vi "Camera_Config_Specific_Attributes.vi"(4 "Crop?":bool, 5 "Camera":T1, 6 "Detect Movement":bool, 8 "error in (no error)":errorcluster, 10 "Refnum in":T2, 11 "input cluster":T3 {"SystemVersion" items=["Standard", "XL"]; "Overlay_Ring" items=["Session Data", "Extended Setup", "Buffer", "Camera", "Dispenser", "Stats", "Connections"]; "Flush Size" min=1; "Dispense Speed" min=1; "Rectangle 2"."Rotation" format="%.2f"; "Rectangle 2"."Left" scale=0.0..1024.0; "Rectangle 2"."Right" scale=0.0..1024.0; "Rectangle 1"."Rotation" format="%.2f"; "Rectangle 1"."Left" scale=0.0..1024.0; "Rectangle 1"."Right" scale=0.0..1024.0; "Max Framerate" min=1; "Overload threshold" min=1; "Image Save Queue Size" min=1; "Image Process Queue Size" min=1; "Empty start" min=1; "Sample size threshold" min=1; "Framerate" min=1; "Light intensity" scale=0.0..100.0}) -> (0 "error out":errorcluster, 3 "Refnum out":T2)   [LabVIEW 2021]
uses:
  <vilib>/userDefined/High Color/IMAQdx.ctl
  controls/Data.ctl
  <vilib>/vision/Image Controls.llb/IMAQ Image.ctl
  Camera_ID.ctl
  <resource>/objmgr/imaqdx.rc
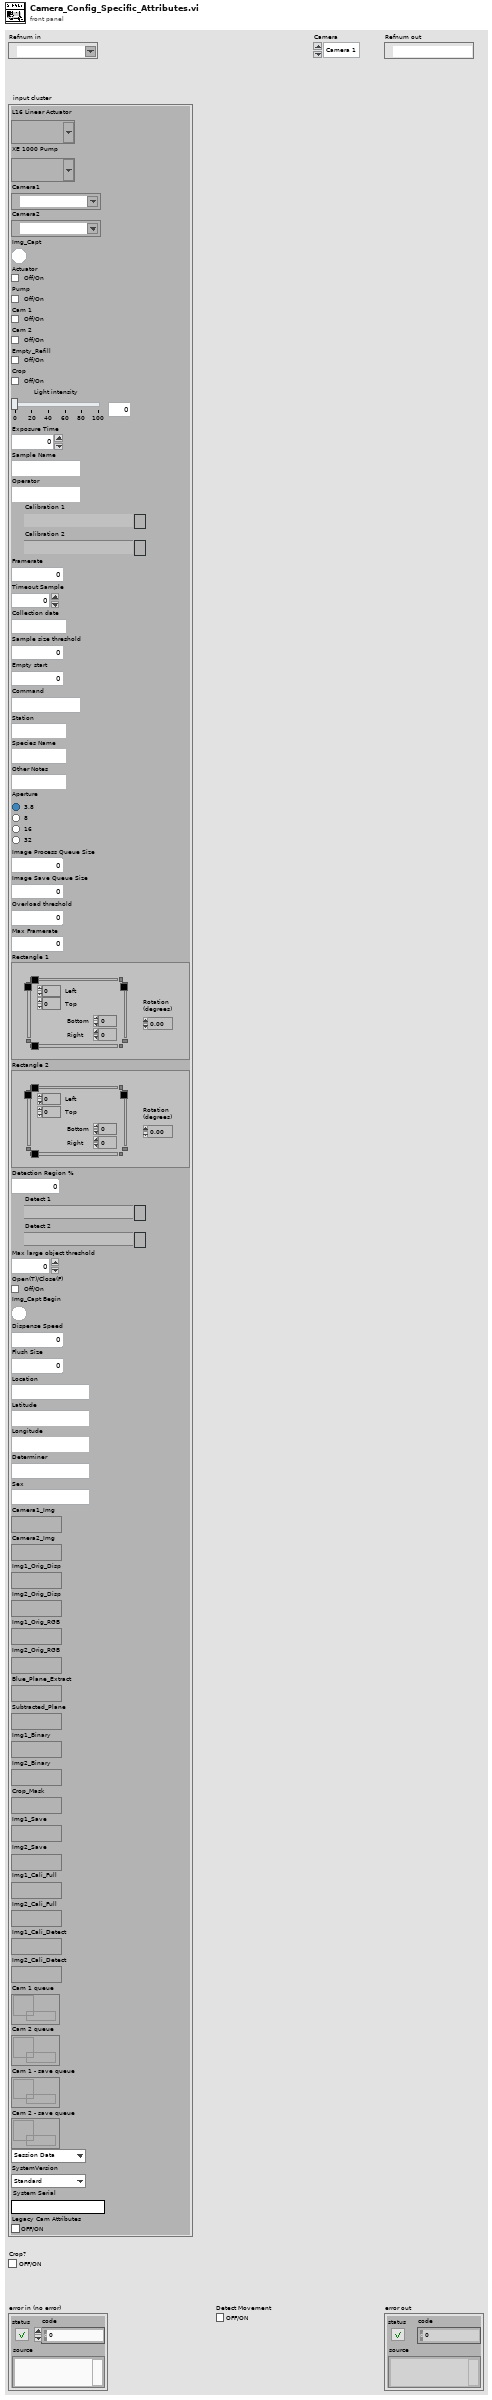
[diagram p1: front panel]
types:
  T1 = typedef "Camera_ID.ctl" = enum16{"Camera 1", "Camera 2"}
  T2 = typedef "IMAQdx.ctl" = refnum<k21>
  T3 = typedef "Data.ctl" = cluster{"L16 Linear Actuator":refnum<visa-resource-name>, "XE 1000 Pump":refnum<visa-resource-name>, "Camera1":T2, "Camera2":T2, "Img_Capt":bool, "Actuator":bool, "Pump":bool, "Cam 1":bool, "Cam 2":bool, "Empty_Refill":bool, "Crop":bool, "Light intensity":i32, "Exposure Time":dbl, "Sample Name":string, "Operator":string, "Calibration 1":path, "Calibration 2":path, "Framerate":i32, "Timeout Sample":i32, "Collection date":string, "Sample size threshold":i32, "Empty start":u32, "Command":string, "Station":string, "Species Name":string, "Other Notes":string, "Aperture":enum32{"Item 0", "Item 1", "Item 2", "Item 3"}, "Image Process Queue Size":i32, "Image Save Queue Size":i32, "Overload threshold":i32, "Max Framerate":i32, "Rectangle 1":T4, "Rectangle 2":T4, "Detection Region %":dbl, "Detect 1":path, "Detect 2":path, "Max large object threshold":i32, "Open(T)/Close(F)":bool, "Img_Capt Begin":bool, "Dispense Speed":i32, "Flush Size":i32, "Location":string, "Latitude":string, "Longitude":string, "Determiner":string, "Sex":string, "Camera1_Img":T5, "Camera2_Img":T5, "Img1_Orig_Disp":T5, "Img2_Orig_Disp":T5, "Img1_Orig_RGB":T5, "Img2_Orig_RGB":T5, "Blue_Plane_Extract":T5, "Subtracted_Plane":T5, "Img1_Binary":T5, "Img2_Binary":T5, "Crop_Mask":T5, "Img1_Save":T5, "Img2_Save":T5, "Img1_Cali_Full":T5, "Img2_Cali_Full":T5, "Img1_Cali_Detect":T5, "Img2_Cali_Detect":T5, "Cam 1 queue":refnum<queue>, "Cam 2 queue":refnum<queue>, "Cam 1 - save queue":refnum<queue>, "Cam 2 - save queue":refnum<queue>, "Overlay_Ring":u16, "SystemVersion":u16, "System Serial":string, "Legacy Cam Attributes":bool}
  T4 = typedef "IMAQ Rectangle" = cluster{"Left":i32, "Top":i32, "Right":i32, "Bottom":i32, "Rotation":dbl}
  T5 = typedef "IMAQ Image.ctl" = refnum<image>
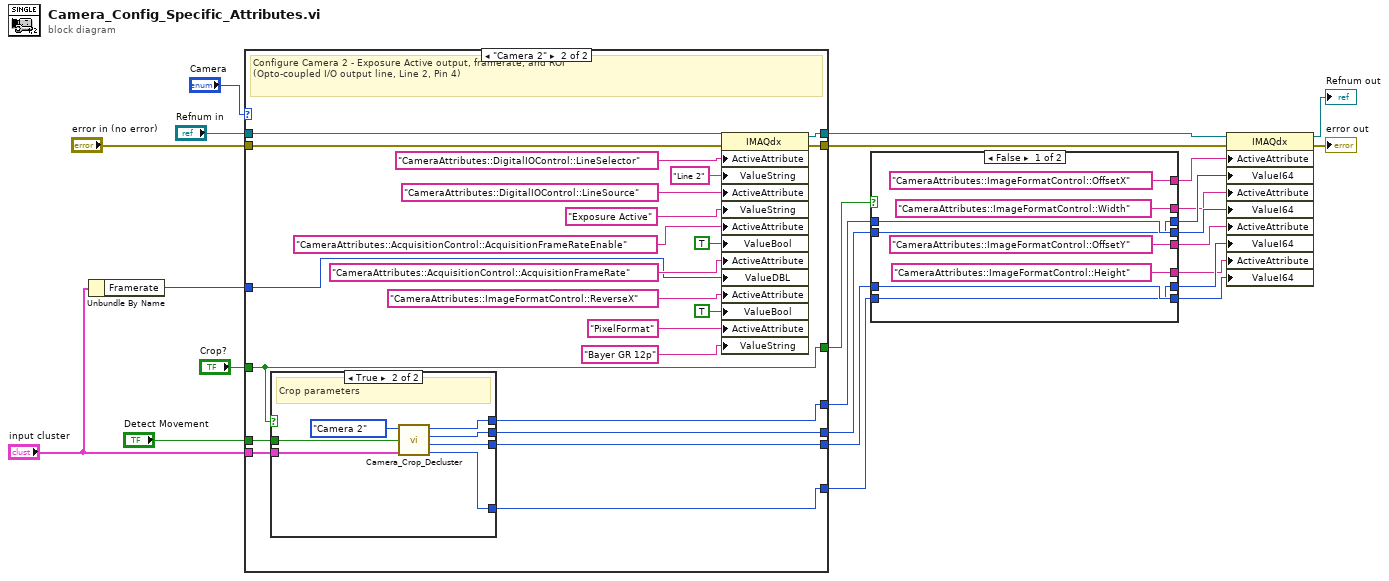
[diagram p0: block diagram]
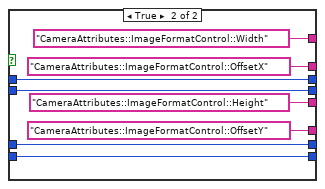
[diagram p2: hidden frame]
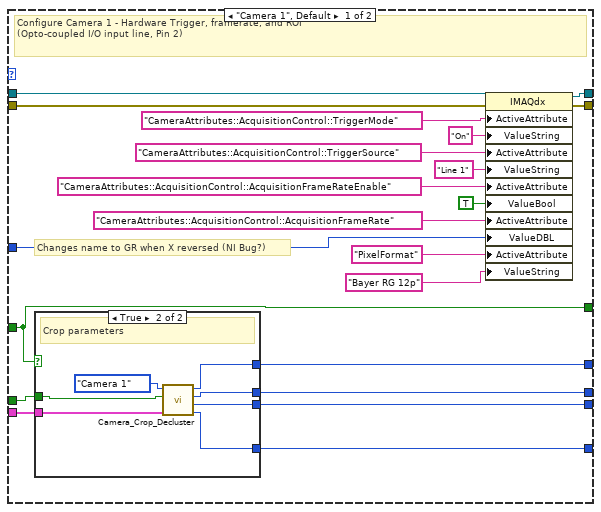
[diagram p3: hidden frame]
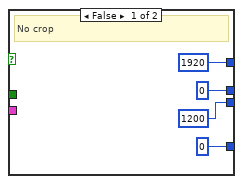
[diagram p4: hidden frame]
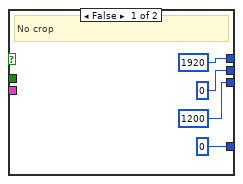
[diagram p5: hidden frame]
diagram:
  n1 = Unbundle By Name("input cluster") -> ("Framerate"=w1:i32)
  n2 = case shown="\"Camera 2\"" "Camera" {
    tunnel: "Refnum in" -> [w45 w66]
    tunnel: [w44 w65] -> w11
    tunnel: [w43 w64] -> w4
    tunnel: w1 -> [w35 w63]
    tunnel: [w33 w79] -> w17
    tunnel: [w34 w78] -> w14
    tunnel: [w31 w76] -> w19
    tunnel: [w32 w77] -> w15
    tunnel: "Crop?" -> [w30 w75]
    tunnel: [w30 w75] -> w12
    tunnel: "input cluster" -> [w29 w74]
    tunnel: "Detect Movement" -> [w28 w73]
    tunnel: "error in (no error)" -> [w27 w59]
    frame "Camera 1", Default {
      # "Changes name to GR when X reversed (NI Bug?)"
      # "Configure Camera 1 - Hardware Trigger, framerate, and ROI \n(Opto-coupled I/O input line, Pin 2)"
      n3 = case shown="True" w30 {
        tunnel: [i64 1920 w55] -> w34
        tunnel: [1200 w53] -> w33
        tunnel: [i64 0 w54] -> w32
        tunnel: [0 w52] -> w31
        tunnel: w29 -> [_ w51]
        tunnel: w28 -> [_ w50]
        frame False {
          # "No crop"
        }
        frame True {
          # "Crop parameters"
          n4 = call "Camera_Crop_Decluster.vi"("input cluster"=w51, "Detect Movement"=w50, "Camera"=Camera_ID."Camera 1") -> ("OffsetY"=w52:i64, "Height"=w53:i64, "OffsetX"=w54:i64, "Width"=w55:i64)  [unwired: 5 in]
        }
      }
      n5 = property class="IMAQdx"(reference=w45, error in=w27, "ActiveAttribute"="CameraAttributes::AcquisitionControl::TriggerMode", "ValueString"="On", "ActiveAttribute"="CameraAttributes::AcquisitionControl::TriggerSource", "ValueString"="Line 1", "ActiveAttribute"="CameraAttributes::AcquisitionControl::AcquisitionFrameRateEnable", "ValueBool"=TRUE, "ActiveAttribute"="CameraAttributes::AcquisitionControl::AcquisitionFrameRate", "ValueDBL"=w35, "ActiveAttribute"="PixelFormat", "ValueString"="Bayer RG 12p") -> (reference out=w44:T2, error out=w43:errorcluster)
    }
    frame "Camera 2" {
      # "Configure Camera 2 - Exposure Active output, framerate, and ROI\n(Opto-coupled I/O output line, Line 2, Pin 4)"
      n6 = case shown="True" w75 {
        tunnel: [i64 1200 w86] -> w79
        tunnel: [i64 1920 w88] -> w78
        tunnel: [i64 0 w87] -> w77
        tunnel: [i64 0 w85] -> w76
        tunnel: w74 -> [_ w90]
        tunnel: w73 -> [_ w84]
        frame False {
          # "No crop"
        }
        frame True {
          # "Crop parameters"
          n7 = call "Camera_Crop_Decluster.vi"("input cluster"=w90, "Detect Movement"=w84, "Camera"=Camera_ID."Camera 2") -> ("OffsetY"=w85:i64, "Height"=w86:i64, "OffsetX"=w87:i64, "Width"=w88:i64)  [unwired: 5 in]
        }
      }
      n8 = property class="IMAQdx"(reference=w66, error in=w59, "ActiveAttribute"="CameraAttributes::DigitalIOControl::LineSelector", "ValueString"="Line 2", "ActiveAttribute"="CameraAttributes::DigitalIOControl::LineSource", "ValueString"="Exposure Active", "ActiveAttribute"="CameraAttributes::AcquisitionControl::AcquisitionFrameRateEnable", "ValueBool"=TRUE, "ActiveAttribute"="CameraAttributes::AcquisitionControl::AcquisitionFrameRate", "ValueDBL"=w63, "ActiveAttribute"="CameraAttributes::ImageFormatControl::ReverseX", "ValueBool"=TRUE, "ActiveAttribute"="PixelFormat", "ValueString"="Bayer GR 12p") -> (reference out=w65:T2, error out=w64:errorcluster)
    }
  }
  n9 = case shown="False" w12 {
    tunnel: ["CameraAttributes::ImageFormatControl::Height" ("ActiveAttribute") "CameraAttributes::ImageFormatControl::OffsetY" ("ActiveAttribute")] -> w5
    tunnel: ["CameraAttributes::ImageFormatControl::OffsetY" ("ActiveAttribute") "CameraAttributes::ImageFormatControl::Height" ("ActiveAttribute")] -> w6
    tunnel: ["CameraAttributes::ImageFormatControl::Width" ("ActiveAttribute") "CameraAttributes::ImageFormatControl::OffsetX" ("ActiveAttribute")] -> w7
    tunnel: ["CameraAttributes::ImageFormatControl::OffsetX" ("ActiveAttribute") "CameraAttributes::ImageFormatControl::Width" ("ActiveAttribute")] -> w8
    tunnel: [w93 w102] -> w13
    tunnel: w14 -> [w94 w102]
    tunnel: w15 -> [w93 w101]
    tunnel: [w94 w101] -> w16
    tunnel: w17 -> [w92 w100]
    tunnel: [w91 w100] -> w18
    tunnel: w19 -> [w91 w99]
    tunnel: [w92 w99] -> w20
    frame False {
    }
    frame True {
    }
  }
  n10 = property class="IMAQdx"(reference=w11, error in=w4, "ActiveAttribute"=w8, "ValueI64"=w13, "ActiveAttribute"=w7, "ValueI64"=w16, "ActiveAttribute"=w6, "ValueI64"=w18, "ActiveAttribute"=w5, "ValueI64"=w20) -> (reference out=→"Refnum out":T2, error out=→"error out":errorcluster)
